vi "Configure Active Trace.vi"(5 "Format":T1, 7 "S parameter":T2(ring), 8 "error in (no error)":errorcluster, 10 "Active Trace":u8=1, 11 "VNA-Ag87xx in":refnum<class "VNA-Ag87xx.lvclass">) -> (0 "error out":errorcluster, 3 "VNA-Ag87xx out":refnum<class "VNA-Ag87xx.lvclass">)   [LabVIEW 2020, in "VNA-Ag87xx.lvclass"]
doc: "Configures the active trace.\nIt creates the trace and sets the S paramert and mode."
uses:
  VNA-Ag87xx.lvclass
  C:/Sandbox/Git_Sandbox/WiSpry Test Framework source code (LV20)/WiSpry Test Framework/Instruments/Instrument.lvclass
  Controls/S parm format enum.ctl
  Instrument.lvclass/Instrument.ctl
  <instrlib>/Agilent 87XX Series/Agilent 87XX Series.lvlib
  Instrument.lvclass
  Vector Network Analyzer.lvclass
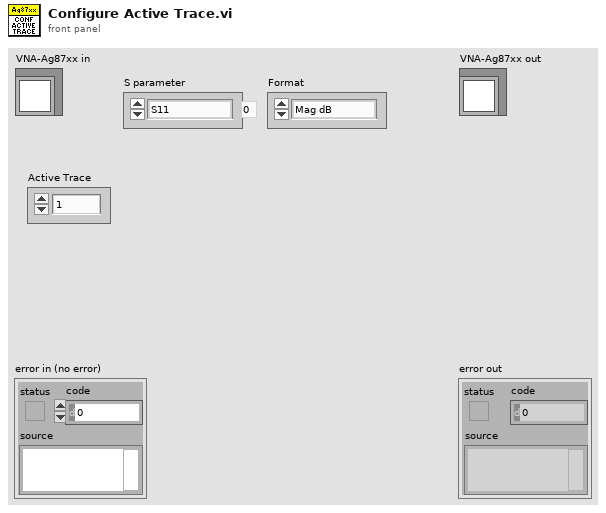
[diagram p1: front panel]
types:
  T1 = typedef "Vector Network Analyzer.lvclass/S parm format enum.ctl" = enum16{"Mag dB", "Mag", "Phase", "Smith", "Real", "Imag", "Group Delay", "SWR"}
  T2 = enum16{"S11", "S21", "S31", "S41", "S22", "S12", "S32", "S42", "S33", "S13", "S23", "S43", "S44", "S14", "S24", "S34"}
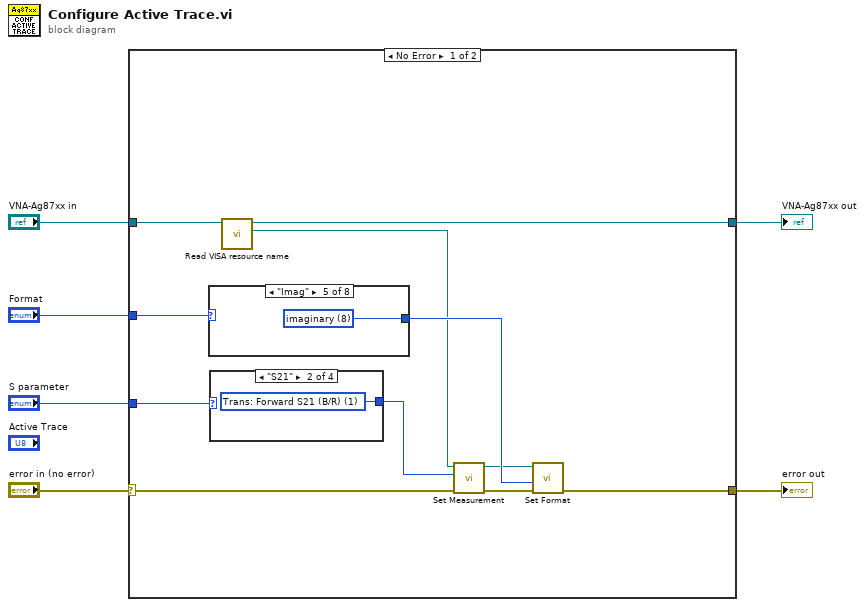
[diagram p0: block diagram]
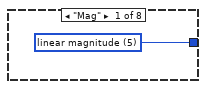
[diagram p2: hidden frame]
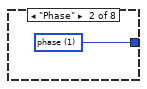
[diagram p3: hidden frame]
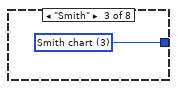
[diagram p4: hidden frame]
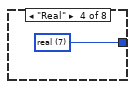
[diagram p5: hidden frame]
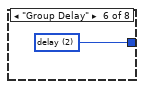
[diagram p6: hidden frame]
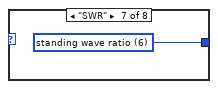
[diagram p7: hidden frame]
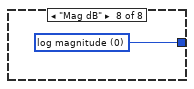
[diagram p8: hidden frame]
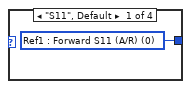
[diagram p9: hidden frame]
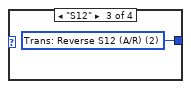
[diagram p10: hidden frame]
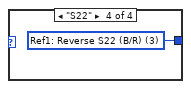
[diagram p11: hidden frame]
diagram:
  n1 = case shown="No Error" "error in (no error)" {
    selector: "error in (no error)" -> [w15 w31]
    tunnel: [w10 w31] -> w5
    tunnel: "VNA-Ag87xx in" -> [w9 w30]
    tunnel: [w8 w30] -> w3
    tunnel: "S parameter" -> [w17 _]
    tunnel: "Format" -> [w14 _]
    frame No Error {
      n2 = case shown="\"Imag\"" w14 {
        tunnel: [w18 w19 w20 w21 w22 w23 w24 w25] -> w13
        frame "Mag" {
          w18 = u16 5 items=["log magnitude", "phase", "delay", "Smith chart", "polar", "linear magnitude", "standing wave ratio", "real", "imaginary"] ("format (0 : log mag)")
        }
        frame "Phase" {
          w19 = u16 1 items=["log magnitude", "phase", "delay", "Smith chart", "polar", "linear magnitude", "standing wave ratio", "real", "imaginary"] ("format (0 : log mag)")
        }
        frame "Smith" {
          w20 = u16 3 items=["log magnitude", "phase", "delay", "Smith chart", "polar", "linear magnitude", "standing wave ratio", "real", "imaginary"] ("format (0 : log mag)")
        }
        frame "Real" {
          w21 = u16 7 items=["log magnitude", "phase", "delay", "Smith chart", "polar", "linear magnitude", "standing wave ratio", "real", "imaginary"] ("format (0 : log mag)")
        }
        frame "Imag" {
          w22 = u16 8 items=["log magnitude", "phase", "delay", "Smith chart", "polar", "linear magnitude", "standing wave ratio", "real", "imaginary"] ("format (0 : log mag)")
        }
        frame "Group Delay" {
          w23 = u16 2 items=["log magnitude", "phase", "delay", "Smith chart", "polar", "linear magnitude", "standing wave ratio", "real", "imaginary"] ("format (0 : log mag)")
        }
        frame "SWR" {
          w24 = u16 6 items=["log magnitude", "phase", "delay", "Smith chart", "polar", "linear magnitude", "standing wave ratio", "real", "imaginary"] ("format (0 : log mag)")
        }
        frame "Mag dB" {
          w25 = u16 0 items=["log magnitude", "phase", "delay", "Smith chart", "polar", "linear magnitude", "standing wave ratio", "real", "imaginary"] ("format (0 : log mag)")
        }
      }
      n3 = case shown="\"S21\"" w17 {
        tunnel: [w26 w27 w28 w29] -> w16
        frame "S11", Default {
          w26 = u16 0 items=["Ref1 : Forward S11 (A/R)", "Trans: Forward S21 (B/R)", "Trans: Reverse S12 (A/R)", "Ref1: Reverse S22 (B/R)", "Analog In, AUX input", "A/R", "B/R", "A/B", "A", "B", "R"] ("measurement (0 : S11)")
        }
        frame "S21" {
          w27 = u16 1 items=["Ref1 : Forward S11 (A/R)", "Trans: Forward S21 (B/R)", "Trans: Reverse S12 (A/R)", "Ref1: Reverse S22 (B/R)", "Analog In, AUX input", "A/R", "B/R", "A/B", "A", "B", "R"] ("measurement (0 : S11)")
        }
        frame "S12" {
          w28 = u16 2 items=["Ref1 : Forward S11 (A/R)", "Trans: Forward S21 (B/R)", "Trans: Reverse S12 (A/R)", "Ref1: Reverse S22 (B/R)", "Analog In, AUX input", "A/R", "B/R", "A/B", "A", "B", "R"] ("measurement (0 : S11)")
        }
        frame "S22" {
          w29 = u16 3 items=["Ref1 : Forward S11 (A/R)", "Trans: Forward S21 (B/R)", "Trans: Reverse S12 (A/R)", "Ref1: Reverse S22 (B/R)", "Analog In, AUX input", "A/R", "B/R", "A/B", "A", "B", "R"] ("measurement (0 : S11)")
        }
      }
      n4 = call "Read VISA resource name.vi"("Instrument in"=w9) -> ("VISA resource name"=w7:refnum<visa-resource-name>, "Instrument out"=w8:refnum<class "VNA-Ag87xx.lvclass">)  [unwired: 9 in]
      n5 = call <instrlib>:"Set Measurement.vi"("error in (no error)"=w15, "measurement (0 : S11)"=w16, "VISA resource name"=w7) -> ("error out"=w12:errorcluster, "VISA resource name out"=w11:refnum<visa-resource-name>)  [unwired: 7 in]
      n6 = call <instrlib>:"Set Format.vi"("error in (no error)"=w12, "format (0 : log mag)"=w13, "VISA resource name"=w11) -> ("error out"=w10:errorcluster)  [unwired: 7 in, 1 out]
    }
    frame Error {
    }
  }
  "error out" <- w5
  "VNA-Ag87xx out" <- w3
